vi "GetConfig.vi"(8 "error in (no error)":errorcluster, 11 "StandardFunction in":refnum<class "StandardFunction.lvclass">) -> (0 "error out":errorcluster, 2 "FunctionConfig":variant, 3 "StandardFunction out":refnum<class "StandardFunction.lvclass">)   [LabVIEW 2018, in "Functions.lvlib" / "StandardFunction.lvclass"]
uses:
  StandardFunction.lvclass
  StandardFunction.lvclass/StandardFunction.ctl
  Accessors/Read StandardWfrms.vi
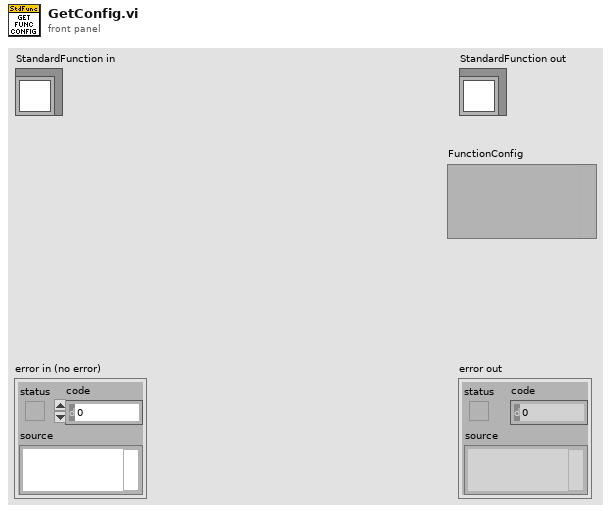
[diagram p1: front panel]
types:
  T1 = typedef "Functions.lvlib/StandardFunction.lvclass/StdWfrms.ctl" = cluster{"Count":u16, "StandardWfrm":T2[]}
  T2 = typedef "Functions.lvlib/StandardFunction.lvclass/StdWfrm.ctl" = cluster{"Amplitude":dbl, "DcOffset":dbl, "DutyCycle":dbl, "Frequency":dbl, "Phase":dbl, "Waveform":enum16{"Sine", "Square", "Triangle", "Ramp Up", "Ramp Down", "DC"}, "Handle":string}
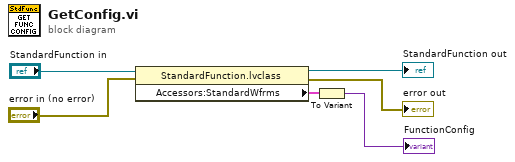
[diagram p0: block diagram]
diagram:
  n1 = property class="StandardFunction.lvclass"(reference="StandardFunction in", error in="error in (no error)") -> (reference out=→"StandardFunction out":refnum<class "StandardFunction.lvclass">, error out=→"error out":errorcluster, "Accessors:StandardWfrms"=w3:T1)
  n2 = To Variant(anything=w3) -> (Variant=→"FunctionConfig":variant)
